vi "Get associated LabVIEW error.vi"(11 "CallResult JSON in":refnum<class "CallResult JSON.lvclass">) -> (2 "LabVIEW Equivalent Error":errorcluster, 3 "CallResult JSON out":refnum<class "CallResult JSON.lvclass">)   [LabVIEW 2020, in "wamplv.lvlib" / "CallResult JSON.lvclass"]
uses:
  CallResult JSON.lvclass
  CallResult JSON.lvclass/CallResult JSON.ctl
  Message loop classes/ErrorOrSuccess JSON/ErrorOrSuccess JSON.lvclass
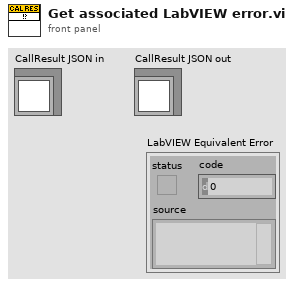
[diagram p1: front panel]
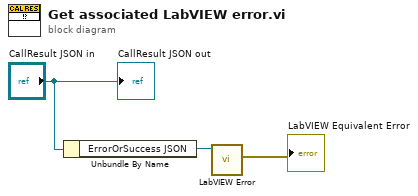
[diagram p0: block diagram]
diagram:
  n1 = Unbundle By Name("CallResult JSON in") -> ("ErrorOrSuccess JSON"=w2:refnum<class "ErrorOrSuccess JSON.lvclass">)
  n2 = call-dynamic "LabVIEW Error.vi"("ErrorOrSuccess JSON in"=w2) -> ("Associated LabVIEW Error"=→"LabVIEW Equivalent Error":errorcluster)  [unwired: 9 in, 1 out]
  "CallResult JSON out" <- "CallResult JSON in"
